vi "BT Rx Test Set BT INSTR TX.vi"(8 "error in (no error)":errorcluster, 10 "niDTS BT.lvlib:niDTS BT INSTR RX":refnum<class "niDTS BT INSTR RX.lvclass">, 11 "niDTS BT Rx Test in":refnum<class "niDTS BT Rx Test.lvclass">) -> (0 "error out":errorcluster, 3 "niDTS BT Rx Test out":refnum<class "niDTS BT Rx Test.lvclass">)   [LabVIEW 2015, in "niDTS BT.lvlib" / "niDTS BT Rx Test.lvclass"]
uses:
  niDTS BT Rx Test.lvclass
  Instrument/INSTR RX/niDTS BT INSTR RX.lvclass
  niDTS BT Rx Test.lvclass/niDTS BT Rx Test.ctl
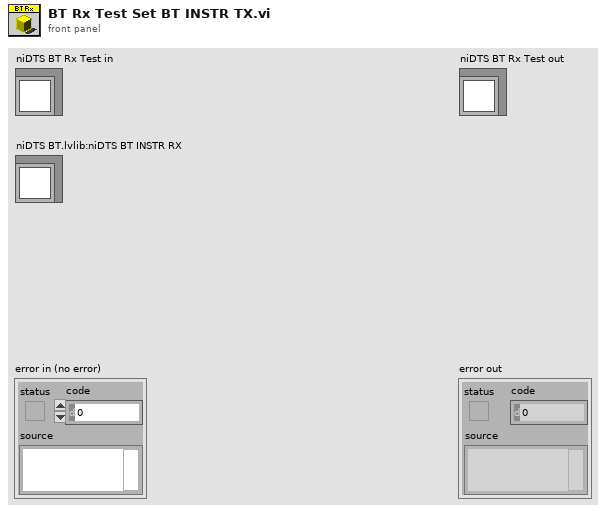
[diagram p1: front panel]
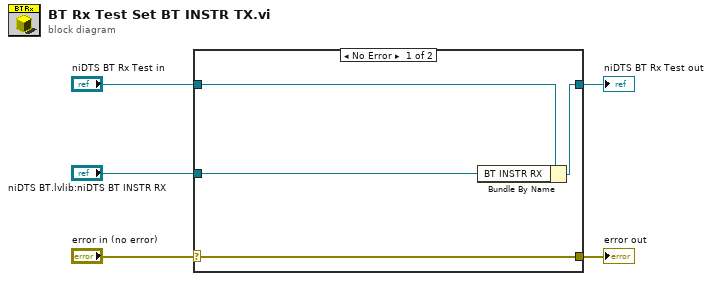
[diagram p0: block diagram]
diagram:
  n1 = case shown="No Error" "error in (no error)" {
    selector: "error in (no error)" -> [w9 w10]
    tunnel: [w9 w10] -> w4
    tunnel: [w7 w11] -> w2
    tunnel: "niDTS BT Rx Test in" -> [w8 w11]
    tunnel: "niDTS BT.lvlib:niDTS BT INSTR RX" -> [w6 _]
    frame No Error {
      n2 = Bundle By Name(cluster=w8, "BT INSTR RX"=w6) -> (w7:refnum<class "niDTS BT Rx Test.lvclass">)
    }
    frame Error {
    }
  }
  "error out" <- w4
  "niDTS BT Rx Test out" <- w2
